vi "Calibration-SaveData.vi"(8 "error in (no error)":errorcluster, 11 "Calibration-RunTest in":refnum<class "Calibration-RunTest.lvclass">) -> (0 "error out":errorcluster, 2 "Cal Finished":bool, 3 "Calibration-RunTest out":refnum<class "Calibration-RunTest.lvclass">)   [LabVIEW 2013, in "Calibration-RunTest.lvclass"]
uses:
  Calibration-RunTest.lvclass
  Calibration-RunTest.lvclass/Calibration-RunTest.ctl
  <vilib>/Utility/file.llb/Write To Spreadsheet File (DBL).vi
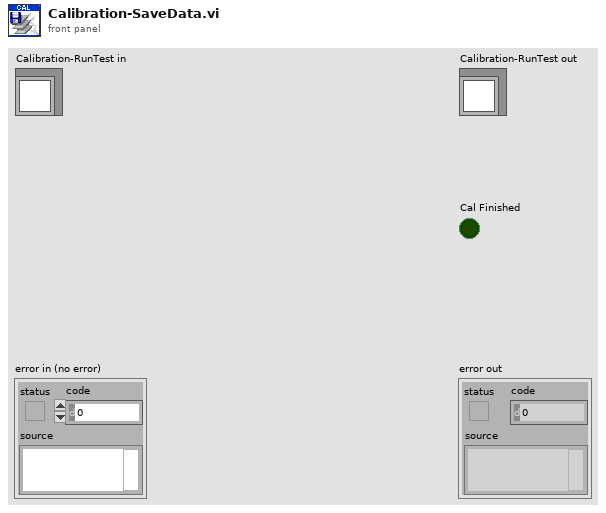
[diagram p1: front panel]
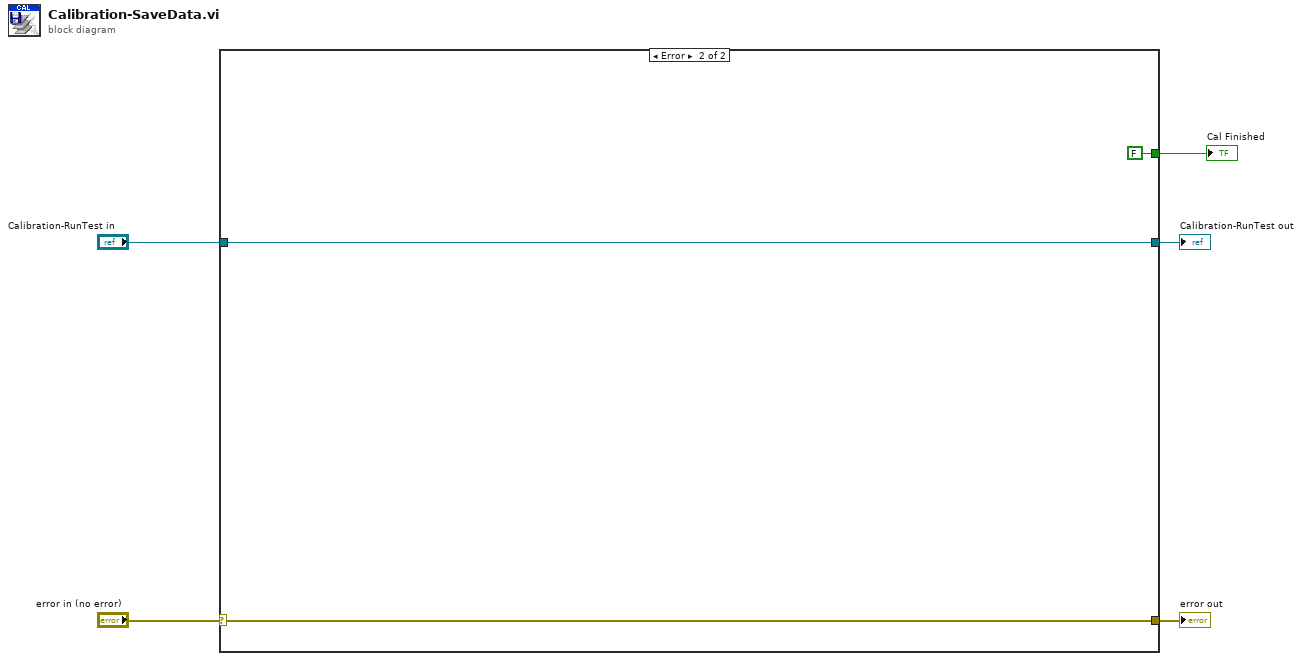
[diagram p0: block diagram]
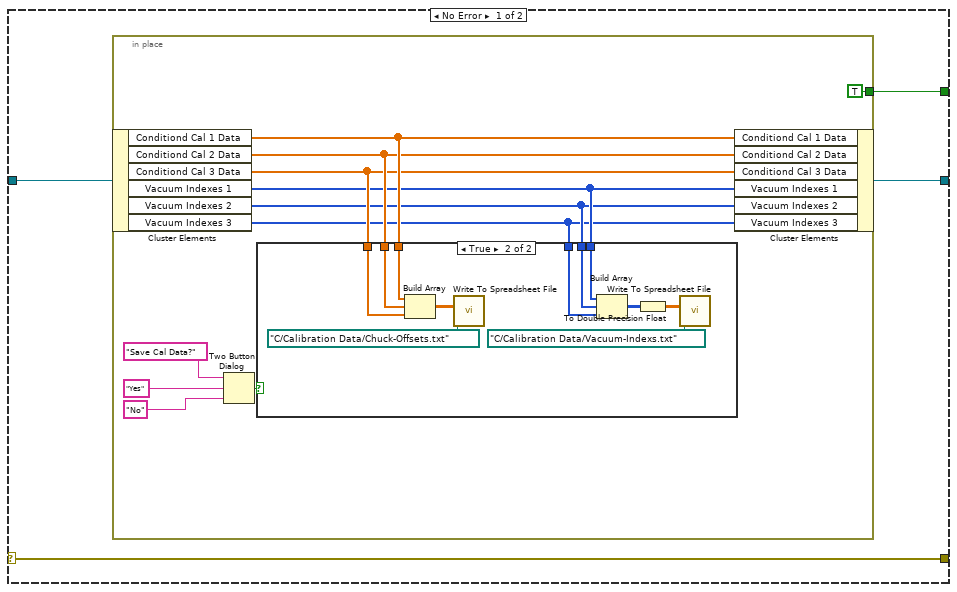
[diagram p2: hidden frame]
diagram:
  n1 = case shown="Error" "error in (no error)" {
    selector: "error in (no error)" -> [w7 w34]
    tunnel: [w7 w34] -> w4
    tunnel: [w8 w33] -> w2
    tunnel: "Calibration-RunTest in" -> [w9 w33]
    tunnel: [w6 FALSE ("Boolean")] -> w1
    frame No Error {
      n2 = in-place {
        in-place-border: [TRUE ("Boolean")] -> w6
        n3 = in-place-cluster #1(w9) -> ("Conditiond Cal 1 Data"=w16:dbl[], "Conditiond Cal 2 Data"=w15:dbl[], "Conditiond Cal 3 Data"=w14:dbl[], "Vacuum Indexes 1"=w13:i32[], "Vacuum Indexes 2"=w12:i32[], "Vacuum Indexes 3"=w11:i32[])
        n4 = Two Button Dialog(message="Save Cal Data?", 1:"No" ("F button name (\"Cancel\")"), 2:"Yes" ("T button name (\"OK\")")) -> (T button?=w17:bool)
        n5 = case shown="True" w17 {
          tunnel: w16 -> [_ w30]
          tunnel: w15 -> [_ w29]
          tunnel: w14 -> [_ w28]
          tunnel: w13 -> [_ w25]
          tunnel: w12 -> [_ w24]
          tunnel: w11 -> [_ w23]
          frame False {
          }
          frame True {
            n6 = Build Array(w30, w29, w28) -> (w27:dbl[][])
            n7 = call-poly <vilib>:"Write To Spreadsheet File.vi"("2D data"=w27, "file path (dialog if empty)"=path "C:/Calibration Data/Chuck-Offsets.txt") -> ()  [unwired: 6 in, 1 out]
            n8 = Build Array(w25, w24, w23) -> (w22:i32[][])
            n9 = To Double Precision Float(number=w22) -> (double precision float=w21:dbl[][])
            n10 = call-poly <vilib>:"Write To Spreadsheet File.vi"("2D data"=w21, "file path (dialog if empty)"=path "C:/Calibration Data/Vacuum-Indexs.txt") -> ()  [unwired: 6 in, 1 out]
          }
        }
        n11 = in-place-cluster #1("Conditiond Cal 1 Data"=w16, "Conditiond Cal 2 Data"=w15, "Conditiond Cal 3 Data"=w14, "Vacuum Indexes 1"=w13, "Vacuum Indexes 2"=w12, "Vacuum Indexes 3"=w11) -> (w8:refnum<class "Calibration-RunTest.lvclass">)
      }
    }
    frame Error {
    }
  }
  "error out" <- w4
  "Calibration-RunTest out" <- w2
  "Cal Finished" <- w1
